vi "LED_top.vi"(5 "FPGA I/O In":refnum<k21>="IO Module\\D0 0", 7 "Testpulser On/Off":bool, 9 "Testpulse Time Delay (20 ns ticks)":u32=15, 10 "Testpulse duration (20 ns ticks)":u32=1, 11 "Address In":u16) -> (0 "Is Test Pulse?":bool, 4 "Randomly generated testpulse separation input (20 ns ticks)":u32=50000)   [LabVIEW 2012]
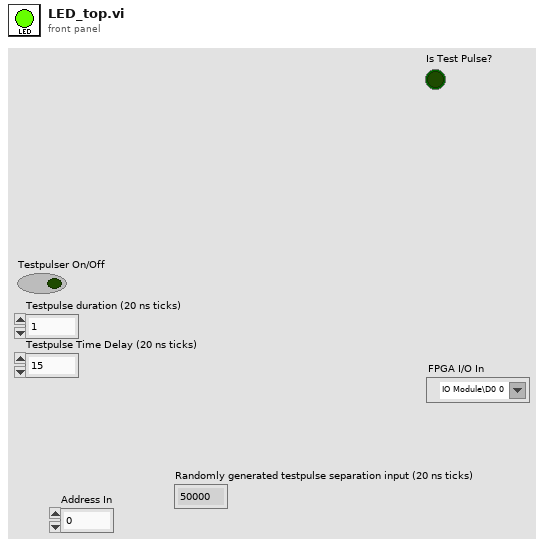
[diagram p1: front panel]
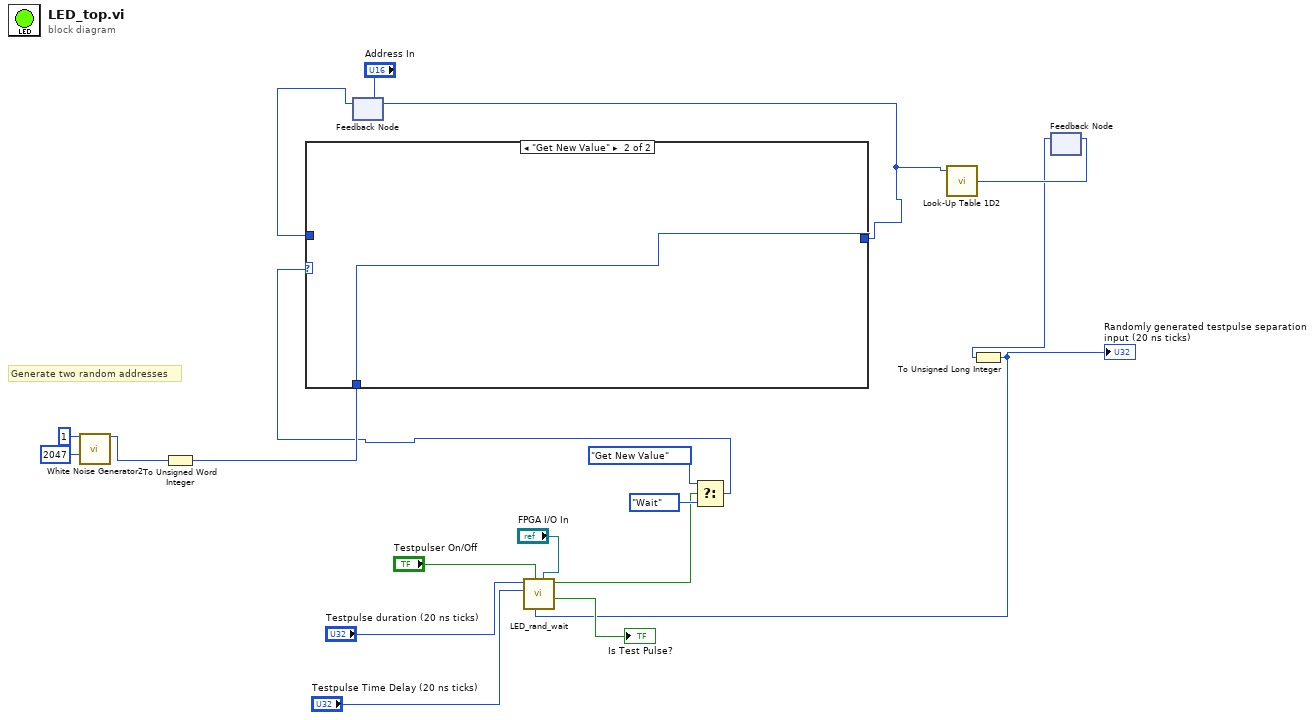
[diagram p0: block diagram]
diagram:
  # "Generate two random addresses"
  n1 = call "White Noise Generator2"("seed"=u32 1, "amplitude"=u16 2047) -> ("white noise out"=w6:i16)  [unwired: 13 in]
  n2 = To Unsigned Word Integer(number=w6) -> (unsigned 16bit integer=w5:u16)
  n3 = feedback #1("Address In") -> (w12:u16)
  n4 = feedback #2() -> (w3:u32)  [unwired: 1 in]
  n5 = To Unsigned Long Integer(number=w3) -> (unsigned 32bit integer=w2:u32)
  "Randomly generated testpulse separation input (20 ns ticks)" <- w2
  n6 = call "LED_rand_wait.vi"("FPGA I/O In"="FPGA I/O In", "Randomly generated testpulse separation input (20 ns ticks)"=w2, "Testpulser On/Off"="Testpulser On/Off", "Testpulse Time Delay (20 ns ticks)"="Testpulse Time Delay (20 ns ticks)", "Testpulse duration (20 ns ticks)"="Testpulse duration (20 ns ticks)") -> ("Is Test Pulse?"=→"Is Test Pulse?":bool, "Get New Value"=w9:bool)  [unwired: 5 in]
  n7 = Select(t=enum16{"Initialize", "Get New Value", "Wait"}."Get New Value", s=w9, f=enum16{"Initialize", "Get New Value", "Wait"}."Wait") -> (s? t:f=w1:enum16{"Initialize", "Get New Value", "Wait"})
  n8 = case shown="\"Get New Value\"" w1 {
    tunnel: w12 -> [w20 _]
    tunnel: w5 -> [_ w21]
    tunnel: [w20 w21] -> w8
    frame "Wait", Default {
    }
    frame "Get New Value" {
    }
  }
  n9 = feedback-in #1(w8) -> ()
  n10 = call "Look-Up Table 1D2"("address"=w8) -> ("data out"=w7:u32)  [unwired: 8 in]
  n11 = feedback-in #2(w7) -> ()
